vi "c_ctre_phoenix6_platform_canbus_is_network_fd.vi"(0 "Numeric":u8, 1 "String 2":string) -> (20 "String":string)   [LabVIEW 2023]
uses:
  <vilib>/Rock Robotics/WPI/ThirdParty/Phoenix-LabVIEW/Controls/DriverLib.ctl
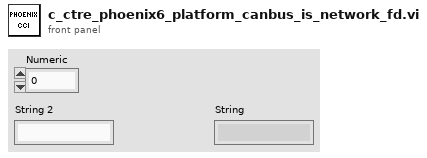
[diagram p1: front panel]
types:
  T1 = typedef "DriverLib.ctl" = path
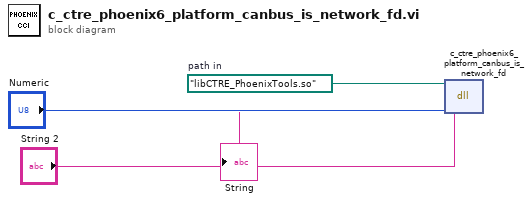
[diagram p0: block diagram]
diagram:
  w4 = T1 path "libCTRE_PhoenixTools.so"  # path in
  n1 = dll-call lib="?" fn="c_ctre_phoenix6_platform_canbus_is_network_fd"(path in=w4, "Numeric", "String 2") -> (→"String":string)  [unwired: 2 in, 2 out]
